vi "Read value.vi"(8 "Error In":errorcluster, 11 "PointerDatatype.lvclass":refnum<class "PointerDatatype.lvclass">) -> (0 "Error Out":errorcluster, 2 "value":string, 3 "PointerDatatype.lvclass 2":refnum<class "PointerDatatype.lvclass">)   [LabVIEW 2014, in "PointerDatatype.lvclass"]
uses:
  PointerDatatype.lvclass
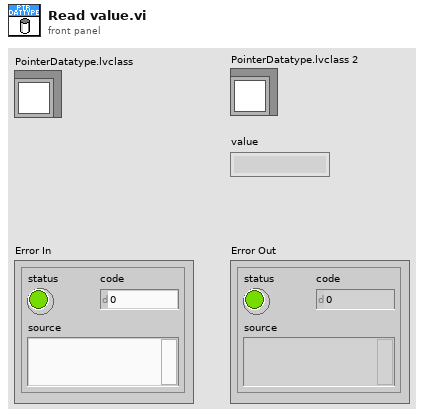
[diagram p1: front panel]
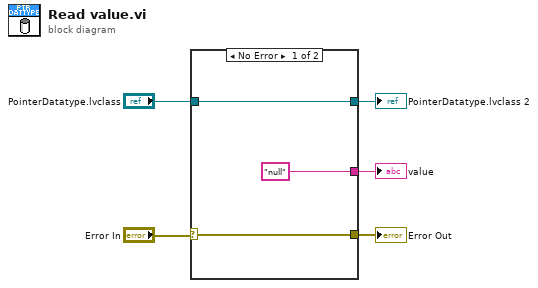
[diagram p0: block diagram]
diagram:
  n1 = case shown="No Error" "Error In" {
    selector: "Error In" -> [w8 w10]
    tunnel: [w8 w10] -> w4
    tunnel: [w7 w9] -> w3
    tunnel: "PointerDatatype.lvclass" -> [w7 w9]
    tunnel: ["null" _] -> w1
    frame No Error {
    }
    frame Error {
    }
  }
  "Error Out" <- w4
  "PointerDatatype.lvclass 2" <- w3
  "value" <- w1
